vi "Initialize.vi"(8 "error in (no error)":errorcluster, 10 "DeviceName":string, 11 "Ztec in":refnum<class "Ztec4611.lvclass">) -> (0 "error out":errorcluster, 1 "new command(s)":string, 2 "DeviceName":string, 3 "Ztec out":refnum<class "Ztec4611.lvclass">)   [LabVIEW 2011, in "Ztec4611.lvclass"]
uses:
  Ztec4611.lvclass
  BaseDriver/BaseDriver.lvclass
  Ztec4611.lvclass/Ztec4611.ctl
panel:
  out "Settings.resourcename":string
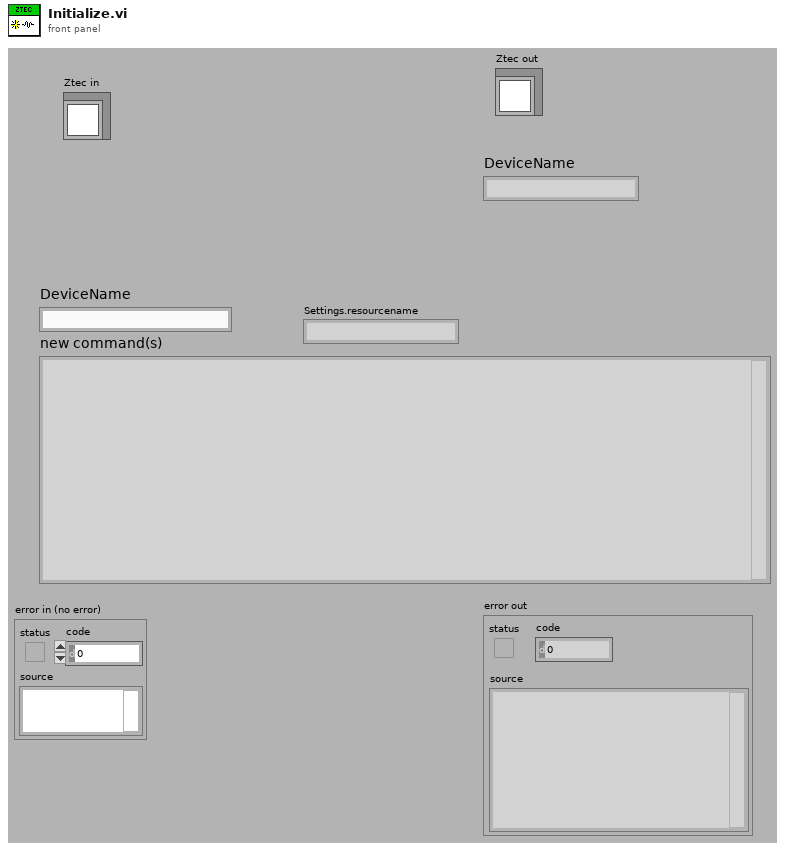
[diagram p1: front panel]
types:
  T1 = typedef "Ztec4611.lvclass/settings_TypDef.ctl" = cluster{"resourcename":string, "timeout":T2, "LocalSavingPath":path, "Save":T3, "probeattenuation":cluster{"Channel0":T2, "Channel1":T2, "Channel2":T2, "Channel3":T2, "Channel4":T2, "Channel5":T2, "Channel6":T2, "Channel7":T2}, "channelenabled":T4, "coupling":cluster{"Channel0":T5, "Channel1":T5, "Channel2":T5, "Channel3":T5, "Channel4":T5, "Channel5":T5, "Channel6":T5, "Channel7":T5}, "impedance":cluster{"Channel0":T6, "Channel1":T6, "Channel2":T6, "Channel3":T6, "Channel4":T6, "Channel5":T6, "Channel6":T6, "Channel7":T6}, "Trigger":cluster{"Slope":T7, "AnalogSource":T8, "Low Level":dbl, "Delay":dbl, "Mode":T9}, "Horizontal":T10, "Names":cluster{"Channel0":string, "Channel1":string, "Channel2":string, "Channel3":string, "Channel4":string, "Channel5":string, "Channel6":string, "Channel7":string}, "verticalrange":cluster{"Channel0":T2, "Channel1":T2, "Channel2":T2, "Channel3":T2, "Channel4":T2, "Channel5":T2, "Channel6":T2, "Channel7":T2}, "offset":cluster{"Channel0":T2, "Channel1":T2, "Channel2":T2, "Channel3":T2, "Channel4":T2, "Channel5":T2, "Channel6":T2, "Channel7":T2}, "Number of channels":dbl, "Method":T11, "LinkedChannel":T13}
  T2 = typedef "numericVariable_TypeDef.ctl" = cluster{"Value":dbl, "Min":dbl, "Max":dbl, "StepSize":dbl, "Tolerance":dbl, "valueactual":dbl}
  T3 = typedef "OnOffTypeDef.ctl" = enum16{"off", "on"}
  T4 = typedef "channelenabled_TypDef.ctl" = cluster{"Channel0":T3, "Channel1":T3, "Channel2":T3, "Channel3":T3, "Channel4":T3, "Channel5":T3, "Channel6":T3, "Channel7":T3}
  T5 = typedef "coupling_Enum_TypDef.ctl" = enum16{"AC", "DC", "Ground"}
  T6 = typedef "impedance_Enum_TypDEf.ctl" = enum16{"1 mega ohm", "<NA>", "50 ohms"}
  T7 = typedef "positive_negatice2_typDef.ctl" = enum16{"Positive", "Negative"}
  T8 = typedef "TriggerSource_TypDef.ctl" = enum16{"Channel 0", "Channel 1", "External TRIG"}
  T9 = typedef "mode_TypDef.ctl" = enum32{"Immediate", "Analog Edge", "Analog Window", "Analog Hysteresis", "Video", "Digital Edge"}
  T10 = typedef "horizontal_TypDef.ctl" = cluster{"min sample rate":dbl, "min record length":i32, "actual record length":i32, "actual sample rate":dbl, "Enforce Realtime":T3}
  T11 = typedef "methodCluster_TypDEf.ctl" = cluster{"Analysis1":T12, "Analysis2":T12, "Analysis3":T12, "Analysis4":T12, "Analysis5":T12, "Analysis6":T12, "Analysis7":T12, "Analysis8":T12, "Analysis9":T12, "Analysis10":T12}
  T12 = typedef "method_TypDef.ctl" = enum16{"n/a", "max", "min", "energy"}
  T13 = typedef "LinkedChannelsCluster_TypDef.ctl" = cluster{"Analysis1":T14, "Analysis2":T14, "Analysis3":T14, "Analysis4":T14, "Analysis5":T14, "Analysis6":T14, "Analysis7":T14, "Analysis8":T14, "Analysis9":T14, "Analysis10":T14}
  T14 = typedef "channels_TypDef.ctl" = enum16{"Channel0", "Channel1", "Channel2", "Channel3", "Channel4", "Channel5", "Channel6", "Channel7", "n/a"}
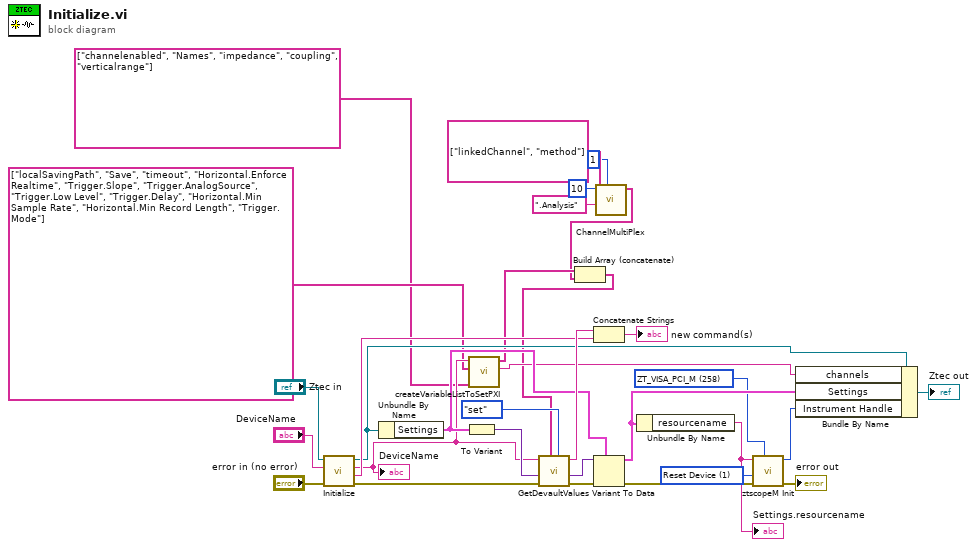
[diagram p0: block diagram]
diagram:
  w8 = 1 items=["Reset Device"=1, "Don't Reset"=0] ("Reset")
  w16 = u16 258 items=["ZT_MCLASS"=2, "ZT_LAN"=4, "ZT_VISA_PCI_M"=258, "ZT_VISA_M"=514] ("Comm Bus")
  n1 = call-parent "Initialize.vi"("error in (no error)"="error in (no error)", "DeviceName"="DeviceName", "BaseDriver in"="Ztec in") -> ("error out"=w21:errorcluster, "new command(s)"=w25:string, "DeviceName"=w17:string, "BaseDriver out"=w24:refnum<class "Ztec4611.lvclass">)  [unwired: 5 in]
  "DeviceName" <- w17
  n2 = Unbundle By Name(w24) -> ("Settings"=w26:T1)
  n3 = To Variant(anything=w26) -> (Variant=w27:variant)
  n4 = call "createVariableListToSetPXI.vi"("set following Variables"=string[] ["channelenabled", "Names", "impedance", "coupling", "verticalrange"] ("set following Variables (empty = all avriables)"), "set following Variables ()"=string[] ["localSavingPath", "Save", "timeout", "Horizontal.Enforce Realtime", "Trigger.Slope", "Trigger.AnalogSource", "Trigger.Low Level", "Trigger.Delay", "Horizontal.Min Sample Rate", "Horizontal.Min Record Length", "Trigger.Mode"] ("set following Variables (empty = all avriables)"), "DeviceName"=w17) -> ("String"=w18:string, "Array"=w4:string[])  [unwired: 7 in]
  n5 = call "ChannelMultiPlex.vi"("start"=1, "string"=".Analysis", "set following Variables"=string[] ["linkedChannel", "method"], "Numeric"=10) -> ("Array"=w3:string[])  [unwired: 6 in, 1 out]
  n6 = Build Array (concatenate)(w4, w3) -> (w2:string[])
  n7 = call "GetDevaultValues.vi"("set or DON'T set"=enum16{"set", "DON'T set"}."set", "set following Variables (empty = all avriables)"=w2, "error in (no error)"=w21, "variant"=w27, "Device Name"=w17) -> ("error out"=w20:errorcluster, "variant out"=w28:variant, "new command(s)"=w29:string)  [unwired: 4 in]
  n8 = Concatenate Strings(w29, w25) -> (→"new command(s)":string)
  n9 = Variant To Data(error in=w20, type=w26, Variant=w28) -> (data=w19:T1, error out=w13:errorcluster)
  n10 = Unbundle By Name(w19) -> ("resourcename"=w15:string)
  "Settings.resourcename" <- w15
  n11 = call "ztscopeM Init.vi"("Resource Name"=w15, "Reset"=w8, "error in"=w13, "Comm Bus"=w16) -> ("Instrument Handle"=w14:i32, "error out"=→"error out":errorcluster)  [unwired: 4 in, 1 out]
  n12 = Bundle By Name(cluster=w24, "channels"=w18, "Settings"=w19, "Instrument Handle"=w14) -> (→"Ztec out":refnum<class "Ztec4611.lvclass">)
